vi "read from connection.vi"(8 "error in":errorcluster, 9 "timeout ms (-1)":i32=-1, 11 "connection in":refnum<class "TCP connection.lvclass">) -> (0 "error out":errorcluster, 1 "valid?":bool, 2 "data message":refnum<class "communicator message.lvclass">, 3 "connection out":refnum<class "TCP connection.lvclass">)   [LabVIEW 2015, in "TCP connection.lvclass"]
uses:
  TCP connection.lvclass
  message/communicator message.lvclass
  TCP connection.lvclass/TCP connection.ctl
  TCP/TCP server.lvclass
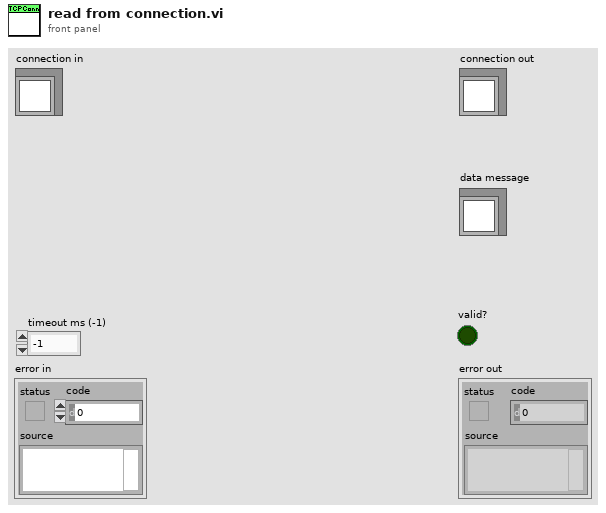
[diagram p1: front panel]
types:
  T1 = enum16{"Standard", "Buffered", "CRLF", "Immediate"}
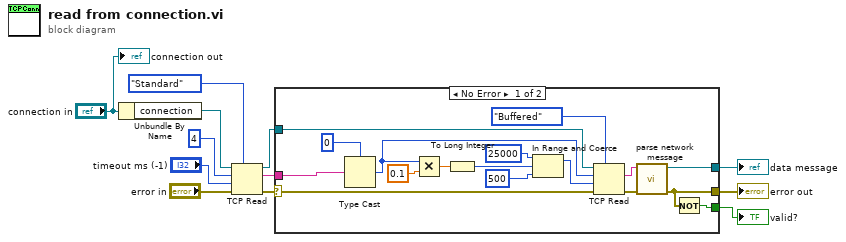
[diagram p0: block diagram]
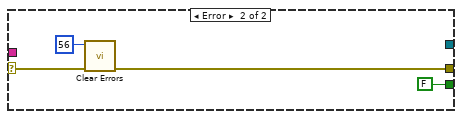
[diagram p2: hidden frame]
diagram:
  n1 = Unbundle By Name("connection in") -> ("connection"=w11:refnum<k5>)
  n2 = TCP Read(connection ID=w11, bytes to read=4, error in (no error)="error in", 7:T1."Standard" ("mode (standard)"), 9:"timeout ms (-1)") -> (connection ID out=w5:refnum<k5>, data out=w6:string, error out=w7:errorcluster)
  n3 = case shown="No Error" w7 {
    selector: w7 -> [w26 w33]
    tunnel: w6 -> [w29 _]
    tunnel: w5 -> [w27 _]
    tunnel: [w15 _] -> w4
    tunnel: [w13 w31] -> w3
    tunnel: [w14 FALSE] -> w2
    frame No Error {
      n4 = Type Cast(type=0, x=w29) -> (*(type *) &x=w21:i32)
      n5 = Multiply(x=w21, y=0.1) -> (x*y=w22:dbl)
      n6 = To Long Integer(number=w22) -> (32bit integer=w17:i32)
      n7 = In Range and Coerce(upper limit=25000 ("timeout ms (25000)"), x=w17, lower limit=500 ("timeout ms (25000)")) -> (coerced(x)=w18:i32)  [unwired: 1 out]
      n8 = TCP Read(connection ID=w27, bytes to read=w21, error in (no error)=w26, 7:T1."Buffered" ("mode (standard)"), 9:w18) -> (data out=w25:string, error out=w16:errorcluster)  [unwired: 1 out]
      n9 = call "parse network message.vi"("error in"=w16, "data"=w25) -> ("error out"=w13:errorcluster, "message"=w15:refnum<class "communicator message.lvclass">)  [unwired: 8 in]
      n10 = Not(x=w13) -> (.not. x?=w14:bool)
    }
    frame Error {
      n11 = call <vilib>:"Clear Errors.vi"("error in (no error)"=w33, "specific error code to clear (0: all)"=56) -> ("error out"=w31:errorcluster)  [unwired: 4 in, 1 out]
    }
  }
  "error out" <- w3
  "data message" <- w4
  "valid?" <- w2
  "connection out" <- "connection in"
